vi "Init Task Data.vi"(9 "DOW":i32, 10 "Task In":T1 {"Action Time" format="%<%H:%M>t"}, 11 "Task Data in":refnum<class "Task Data.lvclass">) -> (3 "Task Data out":refnum<class "Task Data.lvclass">)   [LabVIEW 2012, in "Task Data.lvclass"]
uses:
  Task Data.lvclass
  Type Defs/Timer Control.ctl
  Altitude/Altitude.xctl
  Type Defs/Action Time.ctl
  Mode Control/Mode.xctl
  Task Data.lvclass/Task Data.ctl
  Write Active.vi
  Write Altitude.vi
  Write Act Time.vi
  Write Mode Select.vi
panel:
  # "1"
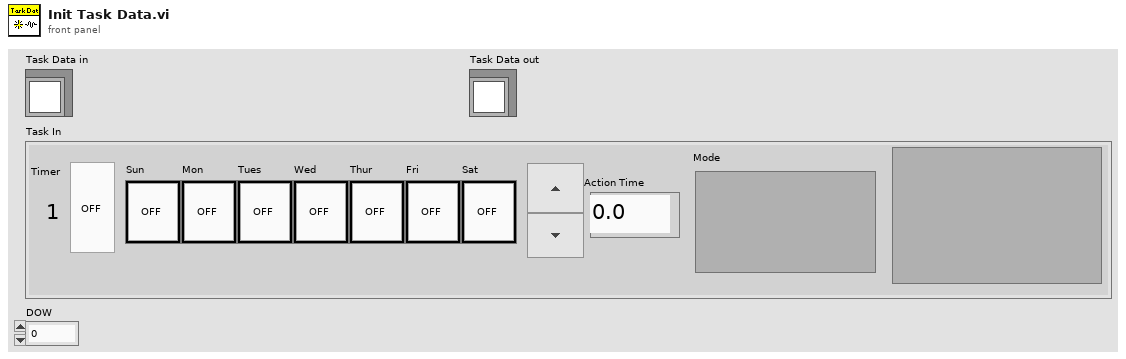
[diagram p1: front panel]
types:
  T1 = typedef "Timer Control.ctl" = cluster{"Sun":bool, "Timer":bool, "Altitude":sgl, "Action Time":T2, "Mon":bool, "Tues":bool, "Wed":bool, "Thur":bool, "Fri":bool, "Sat":bool, "Mode":enum8{"Off", "Stby", "Hold", "Run"}}
  T2 = typedef "Action Time.ctl" = dbl
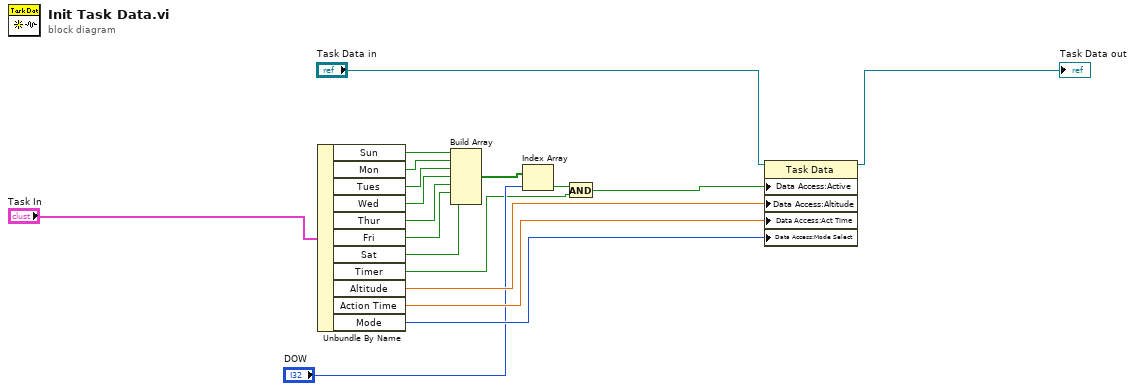
[diagram p0: block diagram]
diagram:
  n1 = Unbundle By Name("Task In") -> ("Sun"=w14:bool, "Mon"=w13:bool, "Tues"=w12:bool, "Wed"=w11:bool, "Thur"=w10:bool, "Fri"=w9:bool, "Sat"=w8:bool, "Timer"=w2:bool, "Altitude"=w17:sgl, "Action Time"=w16:T2, "Mode"=w15:enum8{"Off", "Stby", "Hold", "Run"})
  n2 = Build Array(w14, w13, w12, w11, w10, w9, w8) -> (w7:bool[])
  n3 = Index Array(array=w7, index="DOW") -> (element=w3:bool)
  n4 = And(x=w3, y=w2) -> (x .and. y?=w6:bool)
  n5 = property class="Task Data"(reference="Task Data in", "Data Access:Active"=w6, "Data Access:Altitude"=w17, "Data Access:Act Time"=w16, "Data Access:Mode Select"=w15) -> (reference out=→"Task Data out":refnum<class "Task Data.lvclass">)  [unwired: 1 in, 1 out]
